vi "Measure_Decimate Waveform.vi"(7 "Leftover last":dbl[](array[numeric]), 8 "Error":errorcluster, 9 "Target Sample Rate":dbl=-1.0, 11 "Waveform To Decimate":T1) -> (0 "Error Out":errorcluster, 3 "Waveform Out":T1, 5 "Leftover Out":dbl[](array[numeric]))   [LabVIEW 2020]
uses:
  Universal Controls/Waveform_Data.ctl
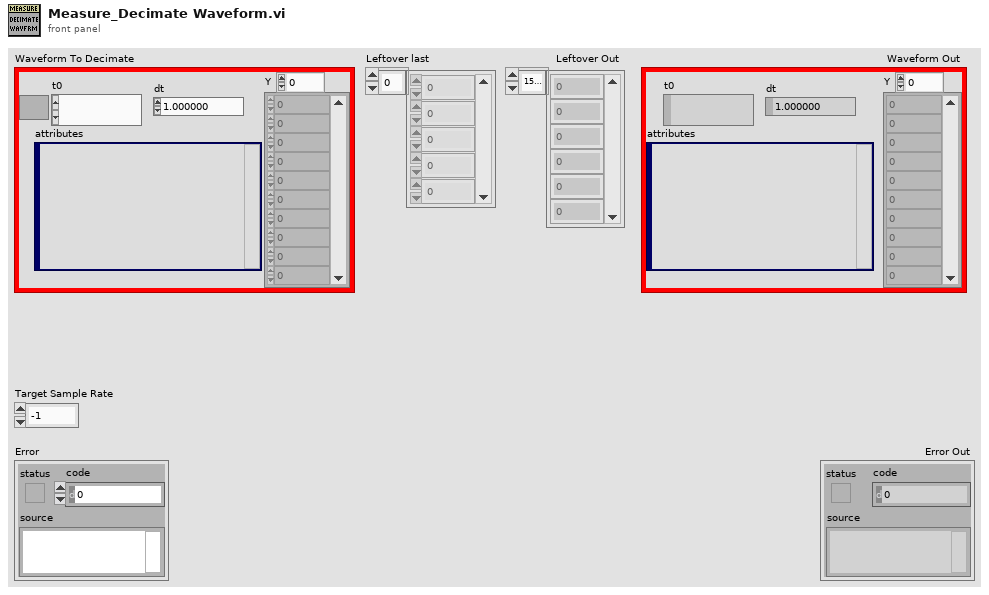
[diagram p1: front panel]
types:
  T1 = typedef "Waveform_Data.ctl" = waveform(dbl)
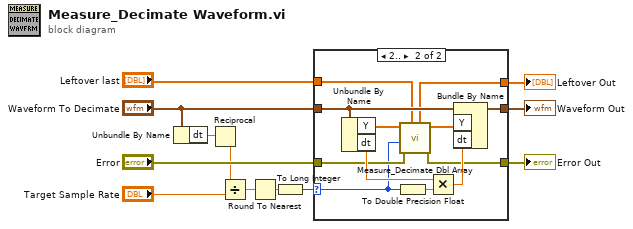
[diagram p0: block diagram]
diagram:
  n1 = Unbundle By Name("Waveform To Decimate") -> ("dt"=w7:dbl)
  n2 = Reciprocal(x=w7) -> (1/x=w3:dbl)
  n3 = Divide(x=w3, y="Target Sample Rate") -> (x/y=w6:dbl)
  n4 = Round To Nearest(number=w6) -> (nearest integer value=w5:dbl)
  n5 = To Long Integer(number=w5) -> (32bit integer=w4:i32)
  n6 = case shown="2.." w4 {
    selector: w4 -> [_ w18]
    tunnel: "Error" -> [w14 w22]
    tunnel: [w14 w21] -> w11
    tunnel: "Waveform To Decimate" -> [w15 w27]
    tunnel: [w15 w26] -> w10
    tunnel: "Leftover last" -> [w13 w20]
    tunnel: [w13 w19] -> w1
    frame ..1 {
    }
    frame 2.. {
      n7 = Unbundle By Name(w27) -> ("Y"=w17:dbl[], "dt"=w25:dbl)
      n8 = To Double Precision Float(number=w18) -> (double precision float=w23:dbl)
      n9 = call "Measure_Decimate Dbl Array.vi"("Leftover Last"=w20, "Error"=w22, "Factor"=w18, "DBL Array"=w17) -> ("Error Out"=w21:errorcluster, "DBL Array Out"=w16:dbl[], "Leftover Out"=w19:dbl[])  [unwired: 5 in]
      n10 = Multiply(x=w25, y=w23) -> (x*y=w24:dbl)
      n11 = Bundle By Name(cluster=w27, "Y"=w16, "dt"=w24) -> (w26:T1)
    }
  }
  "Waveform Out" <- w10
  "Error Out" <- w11
  "Leftover Out" <- w1
